vi "Init_Poly.vi"(1 "2":u8, 2 "1":u8, 3 "0":u8) -> (0 "POLY":u8[](array[numeric]))   [LabVIEW 2022 SP3]
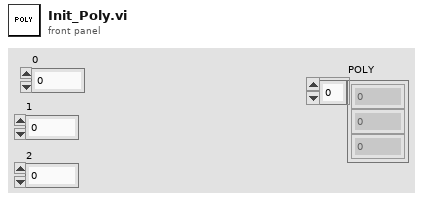
[diagram p1: front panel]
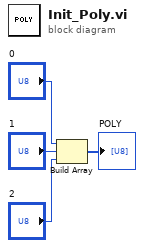
[diagram p0: block diagram]
diagram:
  n1 = Build Array("0", "1", "2") -> (→"POLY":u8[])
